vi "niRFUtil RFHS Channelizer ChannelizerArray CSG.vi"(0 "Channelizer Ref":refnum<data-value>, 1 "Reset":bool, 2 "Benchmark Task":T2, 5 "Data":csg[](array[numeric]), 7 "Data Subset":T1={"Offset"=0, "Length"=-1}, 11 "error in (no error)":errorcluster, 13 "CPU Context":string) -> (4 "Channelizer Ref (out)":refnum<data-value>, 6 "Channel Data":csg[](array[numeric]), 8 "Channel Data Len":u32[](array[numeric]), 15 "error out":errorcluster)   [LabVIEW 2015, in "niRFUtil.lvlib"]
uses:
  niRFUtil.lvlib
  Utilities/Benchmark/niRFUtil RFHS Benchmark Task.ctl
  Utilities/niRFUtil RFHS Util Data Subset.ctl
  Includes/niRFUtil RFHS Channelizer ChannelizerInfo CSG.ctl
  Includes/niRFUtil RFHS Channelizer FilterRef.ctl
  Includes/niRFUtil RFHS Channelizer ChannelizerBufferingMode.ctl
  Utilities/Data FIFO/niRFUtil RFHS FIFO Reference.ctl
  Utilities/Data FIFO/niRFUtil RFHS FIFO.ctl
  Includes/niRFUtil RFHS Channelizer ChannelizerType.ctl
  Includes/niRFUtil RFHS Channelizer ChannelizerFlags.ctl
  Includes/niRFUtil RFHS Channelizer Ref.ctl
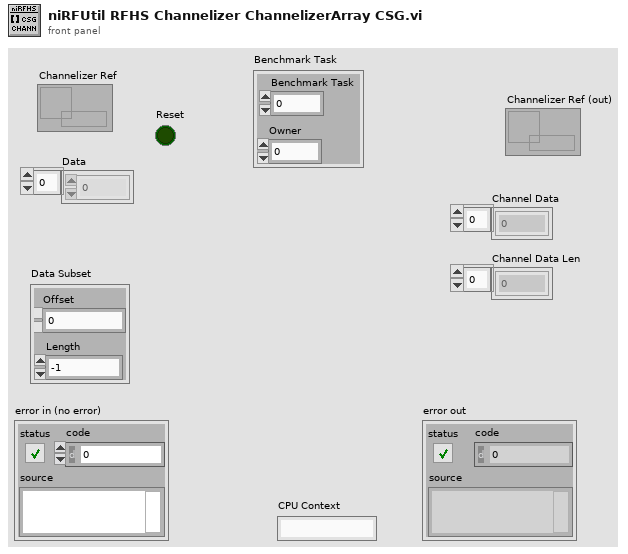
[diagram p1: front panel]
types:
  T1 = typedef "niRFUtil.lvlib/niRFUtil RFHS Util Data Subset.ctl" = cluster{"Offset":i32, "Length":i32}
  T2 = typedef "niRFUtil.lvlib/niRFUtil RFHS Benchmark Task.ctl" = cluster{"Benchmark Task":u64, "Owner":u32}
  T3 = typedef "niRFUtil.lvlib/niRFUtil RFHS Channelizer Ref.ctl" = refnum<data-value>
  T4 = typedef "niRFUtil.lvlib/niRFUtil RFHS Channelizer ChannelizerInfo CSG.ctl" = cluster{"Filter LVRef":T5, "Mode":T6, "History":csg[], "Buffer":csg[], "FIFO":T7, "History Len":u32, "Float Cache":csg[], "Double Cache":cdb[], "Type":T9, "Resample Phase":dbl, "fft1Descriptors":u64[], "fft2Descriptors":u64[], "FFT tBuf":csg[], "guardBandLen":i32, "FFT History":csg[], "FFT History Len":u32, "FFTInitDone":u32, "FFT Filter LVRefs":T5[], "FFT fc Offs":u32[], "fft2Sizes":u32[], "BufferW":u32[], "BufferR":u32[], "Buff Off":u32[], "Phase0 (fshift)":dbl[], "Phase (fshift)":dbl[], "fs phase step":dbl[], "Resample Step":dbl, "Flags":T10, "Reset Cnt":i64, "Filter Pass":u32, "Stages":variant[]}
  T5 = typedef "niRFUtil.lvlib/niRFUtil RFHS Channelizer FilterRef.ctl" = cluster{"Ref":u64, "GUID":u64, "Upsample":i32, "Downsample":i32, "Size":i32, "Num Taps":i32}
  T6 = typedef "niRFUtil.lvlib/niRFUtil RFHS Channelizer ChannelizerBufferingMode.ctl" = enum32{"Unbuffered", "Finite", "Continuous"}
  T7 = typedef "niRFUtil.lvlib/niRFUtil RFHS FIFO Reference.ctl" = cluster{"Read Lock":refnum<data-value>, "Info":T8, "Write Lock":refnum<data-value>}
  T8 = typedef "niRFUtil.lvlib/niRFUtil RFHS FIFO.ctl" = cluster{"ID":u64, "Length":u32}
  T9 = typedef "niRFUtil.lvlib/niRFUtil RFHS Channelizer ChannelizerType.ctl" = enum32{"Auto", "Frequency Shift Only", "Resampler Only"}
  T10 = typedef "niRFUtil.lvlib/niRFUtil RFHS Channelizer ChannelizerFlags.ctl" = u32
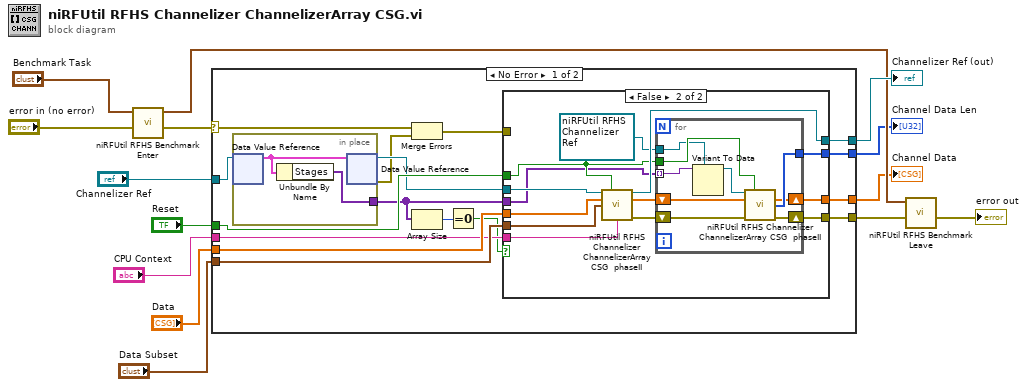
[diagram p0: block diagram]
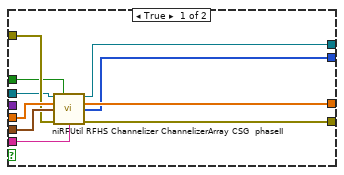
[diagram p2: hidden frame]
diagram:
  n1 = call "niRFUtil RFHS Benchmark Enter.vi"("error in (no error)"="error in (no error)", "Benchmark Task (Parent)"="Benchmark Task") -> ("error out"=w1:errorcluster, "Benchmark Task (Self)"=w5:T2)  [unwired: 8 in]
  n2 = case shown="No Error" w1 {
    selector: w1 -> [w17 w66]
    tunnel: "Data" -> [w30 _]
    tunnel: "Reset" -> [w25 _]
    tunnel: [w15 w66] -> w11
    tunnel: "CPU Context" -> [w26 _]
    tunnel: "Data Subset" -> [w29 _]
    tunnel: "Channelizer Ref" -> [w23 w65]
    tunnel: [w28 w65] -> w6
    tunnel: [w27 _] -> w4
    tunnel: [w24 _] -> w3
    frame No Error {
      n3 = in-place {
        in-place-border: [w63] -> w19
        n4 = in-place-dvr #1(w23) -> (w64:T4)  [unwired: 1 out]
        n5 = Unbundle By Name(w64) -> ("Stages"=w63:variant[])
        n6 = in-place-dvr #1(w64) -> (w22:refnum<data-value>, w18:errorcluster)
      }
      n7 = Merge Errors(w17, w18) -> (w16:errorcluster)
      n8 = Array Size(array=w19) -> (size(s)=w21:i32)
      n9 = Equal To 0?(x=w21) -> (x = 0?=w20:bool)
      n10 = case shown="False" w20 {
        tunnel: w30 -> [w40 w53]
        tunnel: w29 -> [w39 w52]
        tunnel: w16 -> [w38 _]
        tunnel: [w37 w47] -> w15
        tunnel: [w36 w46] -> w28
        tunnel: [w35 w48] -> w27
        tunnel: w26 -> [w34 w44]
        tunnel: w25 -> [w33 w45]
        tunnel: [w32 w49] -> w24
        tunnel: w22 -> [w31 w51]
        tunnel: w19 -> [_ w42]
        frame True {
          n11 = call "niRFUtil RFHS Channelizer ChannelizerArray CSG  phaseII.vi"("Channelizer Ref"=w31, "Reset"=w33, "Data"=w40, "Data Subset"=w39, "error in (no error)"=w38, "CPU Context"=w34) -> ("Channelizer Ref (out)"=w36:refnum<data-value>, "Channel Data"=w35:csg[], "Channel Data Len"=w32:u32[], "error out"=w37:errorcluster)  [unwired: 6 in]
        }
        frame False {
          n12 = call "niRFUtil RFHS Channelizer ChannelizerArray CSG  phaseII.vi"("Channelizer Ref"=w51, "Reset"=w45, "Data"=w53, "Data Subset"=w52, "CPU Context"=w44) -> ("Channelizer Ref (out)"=w46:refnum<data-value>, "Channel Data"=w43:csg[], "error out"=w50:errorcluster)  [unwired: 7 in, 1 out]
          n13 = for {
            tunnel: [w61] -> w49
            tunnel: w45 -> [w58]
            shift-right: [w60] -> w48
            shift-left: w43 -> [w57]
            shift-right: [w59] -> w47
            shift-left: w50 -> [w62]
            tunnel: w42 -> [w56] mode=indexing
            tunnel: T3 refnum ("Channelizer Ref") -> [w55]
            n14 = Variant To Data(type=w55, Variant=w56) -> (data=w54:T3)  [unwired: 1 in, 1 out]
            n15 = call "niRFUtil RFHS Channelizer ChannelizerArray CSG  phaseII.vi"("Channelizer Ref"=w54, "Reset"=w58, "Data"=w57, "error in (no error)"=w62) -> ("Channel Data"=w60:csg[], "Channel Data Len"=w61:u32[], "error out"=w59:errorcluster)  [unwired: 8 in, 1 out]
          }
        }
      }
    }
    frame Error {
    }
  }
  "Channel Data" <- w4
  "Channelizer Ref (out)" <- w6
  "Channel Data Len" <- w3
  n16 = call "niRFUtil RFHS Benchmark Leave.vi"("error in (no error)"=w11, "Benchmark Task Self"=w5) -> ("error out"=→"error out":errorcluster)  [unwired: 8 in, 1 out]
